vi "RT_TVA_time (SubVI).vi"(7 "T [s]":dbl format="%#_13g", 8 "TVA_y_old":dbl, 9 "TVA_p_old":dbl, 10 "TVA_y":dbl, 11 "TVA_p":dbl) -> (3 "TVA_control_time [s]":dbl)   [LabVIEW 2017]
panel:
  out "yaw_time [s]":dbl
  out "pitch_time [s]":dbl
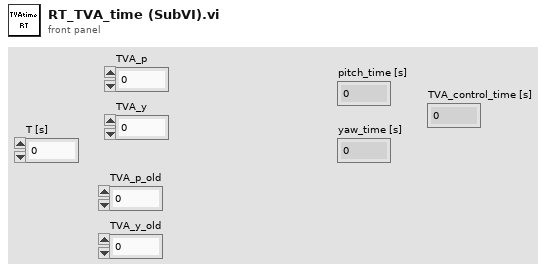
[diagram p1: front panel]
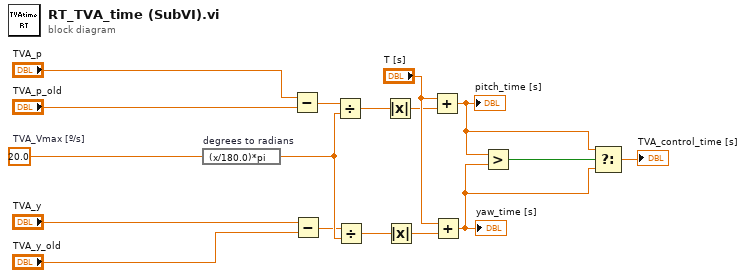
[diagram p0: block diagram]
diagram:
  w5 = 20.0  # TVA_Vmax [º/s]
  n1 = expression code="(x/180.0)*pi" "degrees to radians"(w5) -> (w16:dbl)
  n2 = Subtract(x="TVA_p", y="TVA_p_old") -> (x-y=w8:dbl)
  n3 = Subtract(x="TVA_y", y="TVA_y_old") -> (x-y=w13:dbl)
  n4 = Divide(x=w8, y=w16) -> (x/y=w9:dbl)
  n5 = Divide(x=w13, y=w16) -> (x/y=w12:dbl)
  n6 = Absolute Value(x=w9) -> (abs(x)=w10:dbl)
  n7 = Absolute Value(x=w12) -> (abs(x)=w11:dbl)
  n8 = Add(x="T [s]", y=w10) -> (x+y=w3:dbl)
  "pitch_time [s]" <- w3
  n9 = Add(x="T [s]", y=w11) -> (x+y=w2:dbl)
  "yaw_time [s]" <- w2
  n10 = Greater?(x=w3, y=w2) -> (0:w4:bool)
  n11 = Select(t=w3, s=w4, f=w2) -> (s? t:f=→"TVA_control_time [s]":dbl)
